vi "Get Unit Information.vi"(8 "error in (no error)":errorcluster, 11 "Ethernet_BS1201 in":refnum<class "ENET_BS120x.lvclass">) -> (0 "error out":errorcluster, 1 "Firmware":string, 2 "SerialNumber":string, 3 "Ethernet_BS1201 out":refnum<class "ENET_BS120x.lvclass">, 4 "Calibration Date":string)   [LabVIEW 2021, in "BS120x Driver.lvlib" / "ENET_BS120x.lvclass"]
uses:
  ENET_BS120x.lvclass
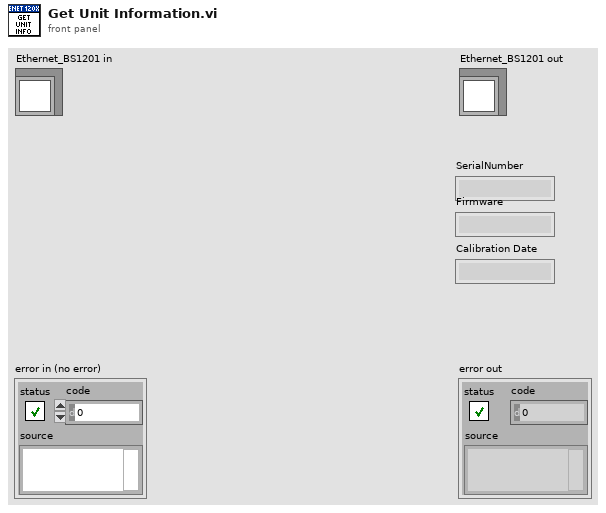
[diagram p1: front panel]
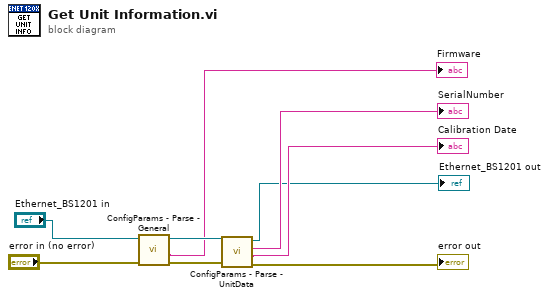
[diagram p0: block diagram]
diagram:
  n1 = call-dynamic "ConfigParams - Parse - General.vi"("error in (no error)"="error in (no error)", "Ethernet in"="Ethernet_BS1201 in") -> ("error out"=w3:errorcluster, "Firmware"=→"Firmware":string, "Ethernet out"=w6:refnum<class "ENET_BS120x.lvclass">)  [unwired: 6 in, 1 out]
  n2 = call-dynamic "ConfigParams - Parse - UnitData.vi"("error in (no error)"=w3, "Ethernet in"=w6) -> ("error out"=→"error out":errorcluster, "Calibration Date"=→"Calibration Date":string, "SerialNumber"=→"SerialNumber":string, "Ethernet out"=→"Ethernet_BS1201 out":refnum<class "ENET_BS120x.lvclass">)  [unwired: 6 in]
